vi "Metadata - table.vi"(8 "error in (no error)":errorcluster, 10 "Database in":string, 11 "mysql in":refnum<class "mysql.lvclass">) -> (0 "error out":errorcluster, 2 "Database metadata":string[][](array[string]), 3 "mysql out":refnum<class "mysql.lvclass">)   [LabVIEW 2020, in "mysql.lvlib" / "mysql.lvclass"]
uses:
  mysql.lvclass
  05ec518d-e1f0-46e6-8c36-3b6b764e9a0e.vi
  <vilib>/Utility/error.llb/Error Cluster From Error Code.vi
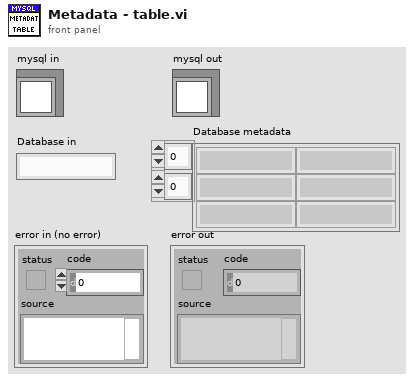
[diagram p1: front panel]
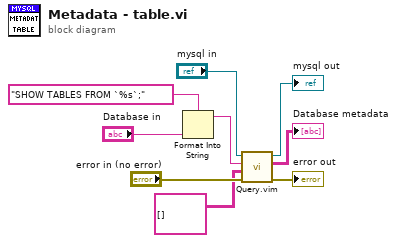
[diagram p0: block diagram]
diagram:
  n1 = Format Into String(format string="SHOW TABLES FROM `%s`;" ("Query string"), "Database in") -> (resulting string=w8:string)  [unwired: 2 in, 1 out]
  n2 = call "Query.vim"("error in (no error)"="error in (no error)", "Type and Default"=string[][] [] ("Database metadata 2"), "Query string"=w8, "IDatabase in"="mysql in") -> ("error out"=→"error out":errorcluster, "Result"=→"Database metadata":string[][], "IDatabase out"=→"mysql out":refnum<class "mysql.lvclass">)  [unwired: 5 in]
